vi "Activate Device.vi"(8 "error in":errorcluster, 10 "DER_Control":T1, 11 "Manual Control in":refnum<class "Manual Control.lvclass">) -> (0 "error out":errorcluster, 3 "Manual Control out":refnum<class "Manual Control.lvclass">)   [LabVIEW 2018, in "Manual Control Actor.lvlib" / "Manual Control.lvclass"]
uses:
  Manual Control.lvclass
  C:/Users/Administrator/Desktop/2018LabVIEW EMS/Device Communication and Control Abstract Actor/Device Communication and Control Abstract/Device Communication and Control Abstract.lvclass
  <vilib>/ORNL/CSEISMIC DDS/CSEISMIC DDS Base/Data Types/DER_Control.ctl
  <vilib>/ORNL/CSEISMIC DDS/CSEISMIC DDS Base/Data Types/Controls/DeviceID.ctl
  Manual Control.lvclass/Manual Control.ctl
  <vilib>/ORNL/CSEISMIC DDS/CSEISMIC DDS Base/Data Types/PCC_Transition.ctl
  <vilib>/ActorFramework/Actor/Actor.lvclass/Actor.ctl
  Device Communication and Control Abstract Actor/Device Communication and Control Abstract/Device Communication and Control Abstract.lvclass/Device Communication and Control Abstract.ctl
  Device Communication and Control Abstract Actor/Device Communication and Control Abstract Messages/Set PCC Transition Msg/Set PCC Transition Msg.lvclass/Set PCC Transition Msg.ctl
  <vilib>/ActorFramework/Message Enqueuer/Message Enqueuer.lvclass/Message Enqueuer.ctl
  <vilib>/ORNL/CSEISMIC DDS/CSEISMIC DDS Base/Data Types/Relay_Control.ctl
  Device Communication and Control Abstract Actor/Device Communication and Control Abstract Messages/Set Relay Control Msg/Set Relay Control Msg.lvclass/Set Relay Control Msg.ctl
  Device Communication and Control Abstract Actor/Device Communication and Control Abstract Messages/Set DER Control Msg/Set DER Control Msg.lvclass/Set DER Control Msg.ctl
  Device Communication and Control Abstract Actor/Device Communication and Control Abstract Messages/Set PCC Transition Msg/Send Set PCC Transition.vi
  <vilib>/ActorFramework/Actor/Read Caller Enqueuer.vi
  Device Communication and Control Abstract Actor/Device Communication and Control Abstract Messages/Set Relay Control Msg/Send Set Relay Control.vi
  Device Communication and Control Abstract Actor/Device Communication and Control Abstract Messages/Set DER Control Msg/Send Set DER Control.vi
  <vilib>/ActorFramework/Message Enqueuer/Enqueue.vi
  Device Communication and Control Abstract Actor/Device Communication and Control Abstract/Device Communication and Control Abstract.lvclass
  C:/Program Files (x86)/National Instruments/LabVIEW 2018/vi.lib/ActorFramework/Actor/Actor.lvclass
  Device Communication and Control Abstract Actor/Device Communication and Control Abstract Messages/Set PCC Transition Msg/Set PCC Transition Msg.lvclass
  C:/Program Files (x86)/National Instruments/LabVIEW 2018/vi.lib/ActorFramework/Message/Message.lvclass
  Device Communication and Control Abstract Actor/Device Communication and Control Abstract Messages/Set Relay Control Msg/Set Relay Control Msg.lvclass
  Device Communication and Control Abstract Actor/Device Communication and Control Abstract Messages/Set DER Control Msg/Set DER Control Msg.lvclass
  <vilib>/ActorFramework/Message Priority Queue/Priority Enqueue.vi
  <vilib>/ORNL/CSEISMIC DDS/CSEISMIC DDS Base/CSEISMIC DDS.lvclass
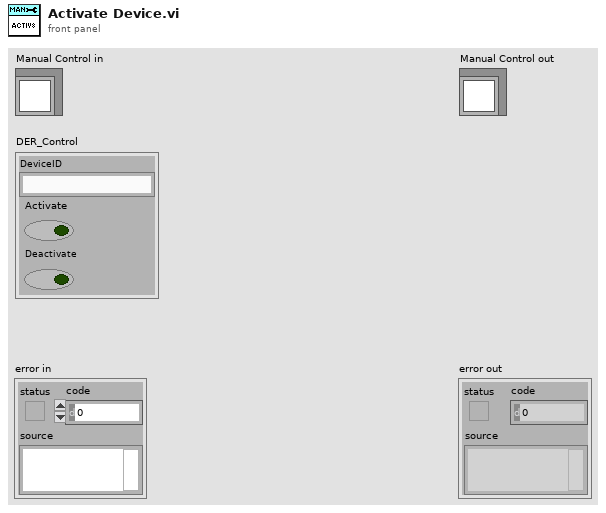
[diagram p1: front panel]
types:
  T1 = typedef "CSEISMIC DDS.lvlib/CSEISMIC DDS.lvclass/DER_Control.ctl" = cluster{"DeviceID":T2, "Activate":bool, "Deactivate":bool}
  T2 = typedef "CSEISMIC DDS.lvlib/CSEISMIC DDS.lvclass/DeviceID.ctl" = string
  T3 = typedef "CSEISMIC DDS.lvlib/CSEISMIC DDS.lvclass/PCC_Transition.ctl" = cluster{"DeviceID":T2, "Island":bool, "Resynchronize":bool}
  T4 = typedef "CSEISMIC DDS.lvlib/CSEISMIC DDS.lvclass/Relay_Control.ctl" = cluster{"DeviceID":T2, "Activate":bool, "Deactivate":bool}
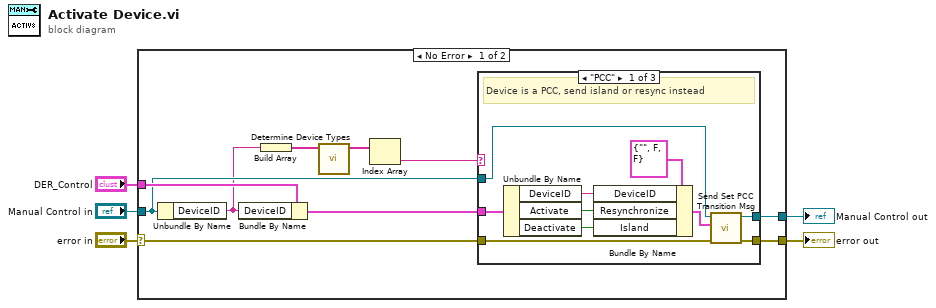
[diagram p0: block diagram]
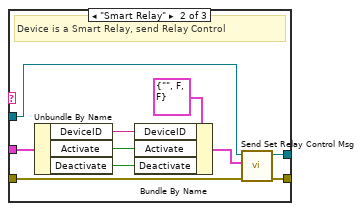
[diagram p2: hidden frame]
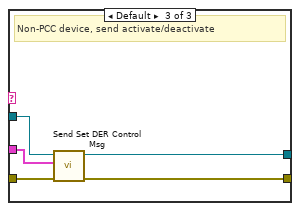
[diagram p3: hidden frame]
diagram:
  n1 = case shown="No Error" "error in" {
    selector: "error in" -> [w11 w42]
    tunnel: [w10 w42] -> w4
    tunnel: [w13 w41] -> w2
    tunnel: "Manual Control in" -> [w14 w41]
    tunnel: "DER_Control" -> [w15 _]
    frame No Error {
      n2 = Unbundle By Name(w14) -> ("DeviceID"=w9:T2)
      n3 = Bundle By Name(cluster=w15, "DeviceID"=w9) -> (w12:T1)
      n4 = Build Array(w9) -> (w8:T2[])
      n5 = call "Determine Device Types.vi"("DeviceIDs"=w8) -> ("Device Classes"=w7:string[])  [unwired: 9 in]
      n6 = Index Array(array=w7) -> (element=w6:string)  [unwired: 1 in]
      n7 = case shown="\"PCC\"" w6 {
        tunnel: w14 -> [w19 w29 w40]
        tunnel: [w18 w28 w39] -> w13
        tunnel: w12 -> [w25 w35 w38]
        tunnel: w11 -> [w16 w26 w37]
        tunnel: [w17 w27 w36] -> w10
        frame "PCC" {
          # "Device is a PCC, send island or resync instead"
          n8 = Unbundle By Name(w25) -> ("DeviceID"=w21:T2, "Activate"=w23:bool, "Deactivate"=w22:bool)
          n9 = Bundle By Name(cluster=T3 {"DeviceID"="", "Island"=FALSE, "Resynchronize"=FALSE} ("PCC_Transition"), "DeviceID"=w21, "Resynchronize"=w23, "Island"=w22) -> (w20:T3)
          n10 = call "Send Set PCC Transition Msg.vi"("error in"=w16, "PCC_Transition"=w20, "SCADA Sub Abstract in"=w19) -> ("error out"=w17:errorcluster, "dup SCADA Sub Abstract"=w18:refnum<class "Manual Control.lvclass">)  [unwired: 7 in]
        }
        frame "Smart Relay" {
          # "Device is a Smart Relay, send Relay Control"
          n11 = Unbundle By Name(w35) -> ("DeviceID"=w31:T2, "Activate"=w33:bool, "Deactivate"=w32:bool)
          n12 = Bundle By Name(cluster=T4 {"DeviceID"="", "Activate"=FALSE, "Deactivate"=FALSE} ("Relay_Control"), "DeviceID"=w31, "Activate"=w33, "Deactivate"=w32) -> (w30:T4)
          n13 = call "Send Set Relay Control Msg.vi"("error in"=w26, "Relay_Control"=w30, "SCADA Sub Abstract in"=w29) -> ("error out"=w27:errorcluster, "dup SCADA Sub Abstract"=w28:refnum<class "Manual Control.lvclass">)  [unwired: 7 in]
        }
        frame Default {
          # "Non-PCC device, send activate/deactivate"
          n14 = call "Send Set DER Control Msg.vi"("error in"=w37, "DER_Control"=w38, "SCADA Sub Abstract in"=w40) -> ("error out"=w36:errorcluster, "dup SCADA Sub Abstract"=w39:refnum<class "Manual Control.lvclass">)  [unwired: 7 in]
        }
      }
    }
    frame Error {
    }
  }
  "error out" <- w4
  "Manual Control out" <- w2
